vi "teleop.vi"   [LabVIEW 2012, in "Joystick Test.lvrbt"]
uses:
  Joystick Test.lvrbt
  <vilib>/NXT/Dual Mode Library/Display/drawText.vi
  <vilib>/NXT/Dual Mode Library/Display/drawNumber.vi
panel:
  # "You may modify the code as needed for your robot. To test this program for an FTC match, open to the Remote Control Editor, select the \"Run Program\" tab, and choose \"Teleop\"."
types:
  T1 = typedef "LVHSConnector.ctl" = refnum<class "BrickReference.lvclass">
  T2 = typedef "FTC ControllerState.ctl" = cluster{"Left X":i8, "Left Y":i8, "Right X":i8, "Right Y":i8, "Button Encoding 9-12":u8, "Button Encoding 1-8":u8, "POV":T3}
  T3 = typedef "FTC POVState.ctl" = i8
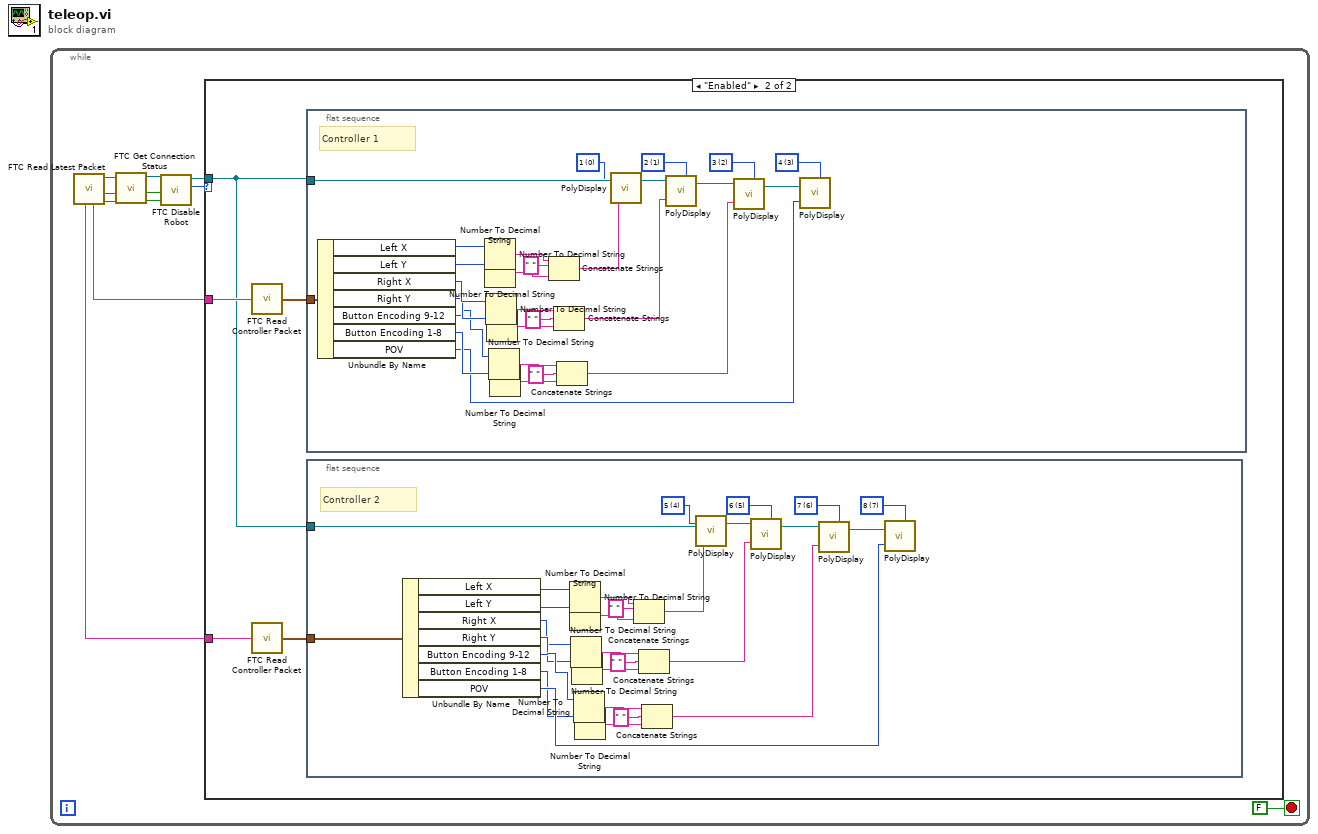
[diagram p0: block diagram]
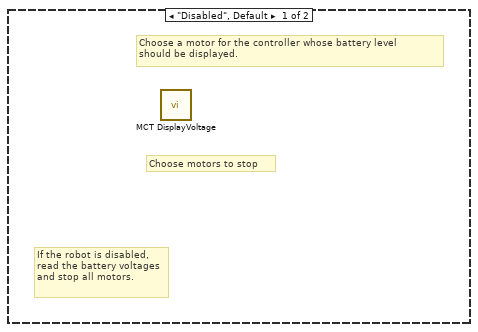
[diagram p2: hidden frame]
diagram:
  n1 = while {
    stop <- FALSE stop-if-true
    n2 = call <vilib>:"FTC Read Latest Packet.vi"() -> ("Packet Received?"=w11:bool, "Stopped?"=w10:bool, "NXT/EV3"=w9:T1, "Controller 1"=w3:string, "Controller 2"=w2:string)  [unwired: 6 in, 1 out]
    n3 = call <vilib>:"FTC Get Connection Status.vi"("Packet Received?"=w11, "Stopped?"=w10, "NXT/EV3"=w9) -> ("Online?"=w8:bool, "Stopped?"=w7:bool, "NXT/EV3"=w6:T1)  [unwired: 5 in]
    n4 = call <vilib>:"FTC Disable Robot.vi"("Online?"=w8, "Stopped?"=w7, "NXT/EV3"=w6) -> ("Enabled?"=w5:enum16{"Disabled", "Enabled"}, "NXT/EV3"=w4:T1)  [unwired: 3 in]
    n5 = case shown="\"Enabled\"" w5 {
      tunnel: w4 -> [_ w12]
      tunnel: w3 -> [_ w16]
      tunnel: w2 -> [_ w13]
      frame "Disabled", Default {
        # "Choose motors to stop"
        # "Choose a motor for the controller whose battery level \nshould be displayed."
        # "If the robot is disabled, read the battery voltages and stop all motors."
        n6 = call <vilib>:"MCT DisplayVoltage.vi"() -> ()  [unwired: 11 in, 1 out]
      }
      frame "Enabled" {
        n7 = call <vilib>:"FTC Read Controller Packet.vi"("Packet"=w16) -> ("Controller State"=w14:T2)  [unwired: 4 in]
        n8 = call <vilib>:"FTC Read Controller Packet.vi"("Packet"=w13) -> ("Controller State"=w15:T2)  [unwired: 4 in]
        n9 = flat-sequence {
          tunnel: w14 -> [w45]
          tunnel: w12 -> [w72]
          frame #0 {
            w65 = i16 3 items=["1", "2", "3", "4", "5", "6", "7", "8", "9", "10", "11", "12"] ("Line")
            w66 = i16 2 items=["1", "2", "3", "4", "5", "6", "7", "8", "9", "10", "11", "12"] ("Line")
            w67 = i16 1 items=["1", "2", "3", "4", "5", "6", "7", "8", "9", "10", "11", "12"] ("Line")
            w71 = i16 0 items=["1", "2", "3", "4", "5", "6", "7", "8", "9", "10", "11", "12"] ("Line")
            # "Controller 1"
            n10 = Unbundle By Name(w45) -> ("Left X"=w64:i8, "Left Y"=w59:i8, "Right X"=w54:i8, "Right Y"=w53:i8, "Button Encoding 9-12"=w49:u8, "Button Encoding 1-8"=w48:u8, "POV"=w46:T3)
            n11 = Number To Decimal String(number=w64) -> (decimal integer string=w63:string)  [unwired: 1 in]
            n12 = Number To Decimal String(number=w59) -> (decimal integer string=w62:string)  [unwired: 1 in]
            n13 = Number To Decimal String(number=w54) -> (decimal integer string=w56:string)  [unwired: 1 in]
            n14 = Number To Decimal String(number=w53) -> (decimal integer string=w57:string)  [unwired: 1 in]
            n15 = Number To Decimal String(number=w49) -> (decimal integer string=w52:string)  [unwired: 1 in]
            n16 = Number To Decimal String(number=w48) -> (decimal integer string=w51:string)  [unwired: 1 in]
            n17 = Concatenate Strings(w63, " " ("string"), w62) -> (w60:string)
            n18 = Concatenate Strings(w56, " " ("string"), w57) -> (w55:string)
            n19 = Concatenate Strings(w52, " " ("string"), w51) -> (w47:string)
            n20 = call-poly <vilib>:"PolyDisplay.vi"("Text"=w60, "NXT/EV3"=w72, "Line"=w71) -> ("NXT/EV3"=w70:T1)  [unwired: 1 in]
            n21 = call-poly <vilib>:"PolyDisplay.vi"("Text"=w55, "NXT/EV3"=w70, "Line"=w67) -> ("NXT/EV3"=w69:T1)  [unwired: 1 in]
            n22 = call-poly <vilib>:"PolyDisplay.vi"("Text"=w47, "NXT/EV3"=w69, "Line"=w66) -> ("NXT/EV3"=w68:T1)  [unwired: 1 in]
            n23 = call-poly <vilib>:"PolyDisplay.vi"("number"=w46, "NXT/EV3"=w68, "Line"=w65) -> ()  [unwired: 1 in, 1 out]
          }
        }
        n24 = flat-sequence {
          tunnel: w15 -> [w17]
          tunnel: w12 -> [w18]
          frame #0 {
            w25 = i16 7 items=["1", "2", "3", "4", "5", "6", "7", "8", "9", "10", "11", "12"] ("Line")
            w24 = i16 6 items=["1", "2", "3", "4", "5", "6", "7", "8", "9", "10", "11", "12"] ("Line")
            w23 = i16 5 items=["1", "2", "3", "4", "5", "6", "7", "8", "9", "10", "11", "12"] ("Line")
            w19 = i16 4 items=["1", "2", "3", "4", "5", "6", "7", "8", "9", "10", "11", "12"] ("Line")
            # "Controller 2"
            n25 = Unbundle By Name(w17) -> ("Left X"=w26:i8, "Left Y"=w31:i8, "Right X"=w36:i8, "Right Y"=w37:i8, "Button Encoding 9-12"=w41:u8, "Button Encoding 1-8"=w42:u8, "POV"=w44:T3)
            n26 = Number To Decimal String(number=w26) -> (decimal integer string=w27:string)  [unwired: 1 in]
            n27 = Number To Decimal String(number=w31) -> (decimal integer string=w28:string)  [unwired: 1 in]
            n28 = Number To Decimal String(number=w36) -> (decimal integer string=w34:string)  [unwired: 1 in]
            n29 = Number To Decimal String(number=w37) -> (decimal integer string=w33:string)  [unwired: 1 in]
            n30 = Number To Decimal String(number=w41) -> (decimal integer string=w38:string)  [unwired: 1 in]
            n31 = Number To Decimal String(number=w42) -> (decimal integer string=w39:string)  [unwired: 1 in]
            n32 = Concatenate Strings(w27, " " ("string"), w28) -> (w30:string)
            n33 = Concatenate Strings(w34, " " ("string"), w33) -> (w35:string)
            n34 = Concatenate Strings(w38, " " ("string"), w39) -> (w43:string)
            n35 = call-poly <vilib>:"PolyDisplay.vi"("Text"=w30, "NXT/EV3"=w18, "Line"=w19) -> ("NXT/EV3"=w20:T1)  [unwired: 1 in]
            n36 = call-poly <vilib>:"PolyDisplay.vi"("Text"=w35, "NXT/EV3"=w20, "Line"=w23) -> ("NXT/EV3"=w21:T1)  [unwired: 1 in]
            n37 = call-poly <vilib>:"PolyDisplay.vi"("Text"=w43, "NXT/EV3"=w21, "Line"=w24) -> ("NXT/EV3"=w22:T1)  [unwired: 1 in]
            n38 = call-poly <vilib>:"PolyDisplay.vi"("number"=w44, "NXT/EV3"=w22, "Line"=w25) -> ()  [unwired: 1 in, 1 out]
          }
        }
      }
    }
  }
